vi "Acquire Data.vi"() -> ()   [LabVIEW 2020]
uses:
  states.ctl
  <vilib>/FPGAPlugInAG/cRIO-9066/niLvFpga_Open_cRIO-9066.vi
  <vilib>/rvi/interface/common/dynamic/niFpgaDynamicAddResources.vi
  <vilib>/Utility/error.llb/Error Cluster From Error Code.vi
  <vilib>/rvi/errors/niLvFpgaAdjustHostInterfaceError.vi
  <vilib>/rvi/interface/nirviOpenFPGA/nirviOpenFPGA.xnode
  FPGA Bitfiles/realcrioexample_FPGATarget_GetcRIOTemp_ZmXcEI1H0PA.lvbitx
  FPGA/Get cRIO Temp.vi
  <vilib>/rvi/interface/nirviReadWriteControl/nirviReadWriteControl.xnode
  NiFpgaLv.dll
  <vilib>/rvi/interface/Simulation/niFpgaSimulationCallBeginRW.vi
panel:
  out "Chassis Temperature":i16
  out "Chassis Temp History":i16[](array[numeric])
  in  "shutdown":bool
  in  "save to txt":bool
  in  "grab cRIO data":bool
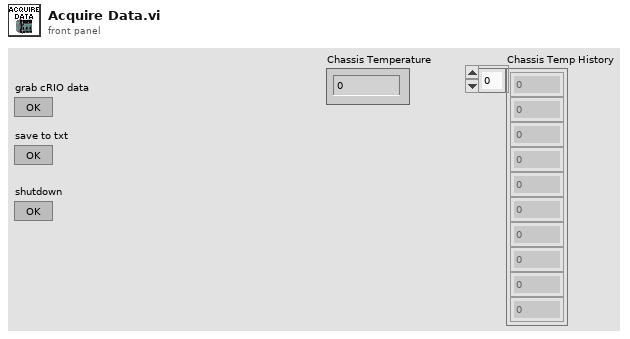
[diagram p1: front panel]
types:
  T1 = typedef "states.ctl" = enum16{"Start", "Save Data", "Shutdown"}
  T2 = enum16{"open", "replace", "create", "open or create", "replace or create", "replace or create with confirmation"}
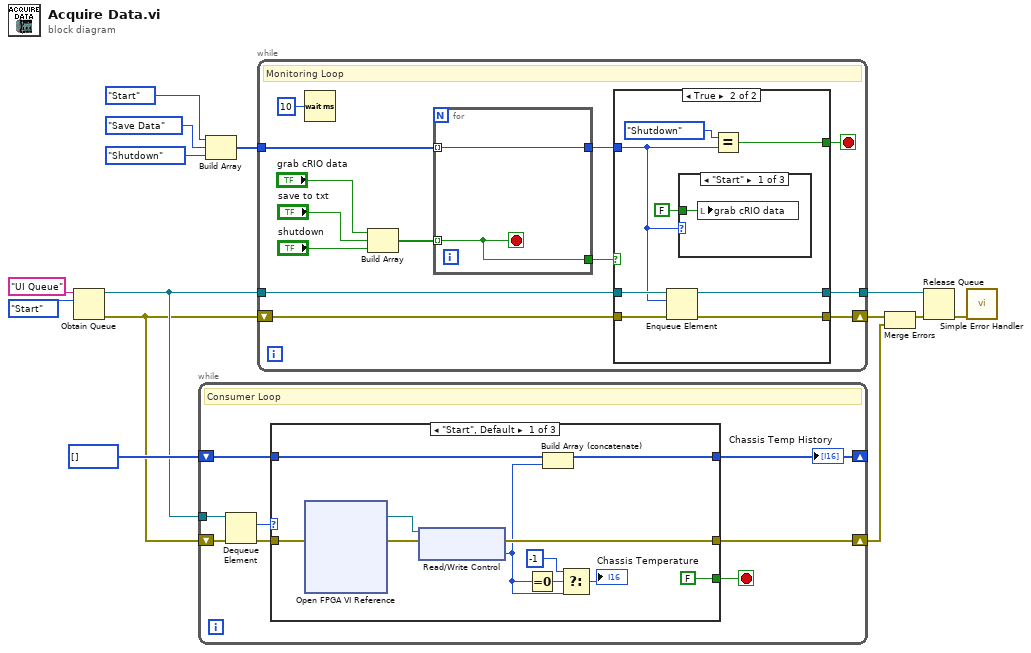
[diagram p0: block diagram]
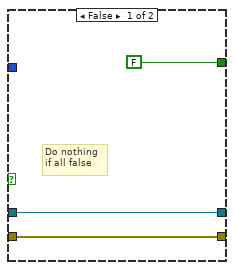
[diagram p2: hidden frame]
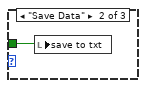
[diagram p3: hidden frame]
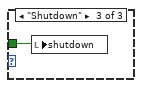
[diagram p4: hidden frame]
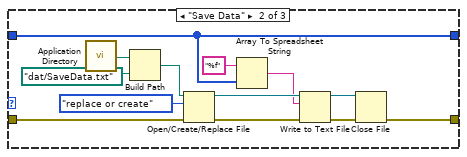
[diagram p5: hidden frame]
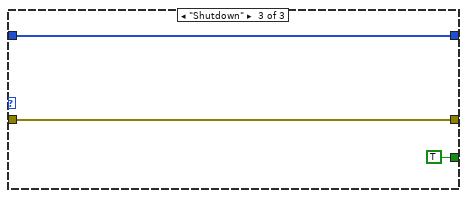
[diagram p6: hidden frame]
diagram:
  n1 = Obtain Queue(name (unnamed)="UI Queue", element data type=states."Start") -> (queue out=w5:refnum<queue>, error out=w4:errorcluster)  [unwired: 3 in, 1 out]
  n2 = while {
    tunnel: w5 -> [w22]
    shift-right: [w18] -> _
    shift-left: i16[] [] -> [w17]
    shift-right: [w15] -> w10
    shift-left: w4 -> [w21]
    stop <- w19 stop-if-true
    # "Consumer Loop"
    n3 = Dequeue Element(queue=w22, error in (no error)=w21) -> (element=w20:T1, error out=w16:errorcluster)  [unwired: 1 in, 2 out]
    n4 = case shown="\"Start\", Default" w20 {
      tunnel: [FALSE _ TRUE] -> w19
      tunnel: [w27 w45 w49] -> w18
      tunnel: w17 -> [w28 w45 w49]
      tunnel: w16 -> [w32 w35 w48]
      tunnel: [w29 w34 w48] -> w15
      frame "Start", Default {
        n5 = xnode "Open FPGA VI Reference"("error in"=w32) -> ("FPGA VI Reference Out"=w31:refnum<k20>, "error out"=w30:errorcluster)  [unwired: 1 in]
        n6 = xnode "Read/Write Control"("FPGA VI Reference In"=w31, "error in"=w30) -> ("error out"=w29:errorcluster, "chassis temp"=w23:i16)  [unwired: 1 out]
        n7 = Equal To 0?(x=w23) -> (x = 0?=w26:bool)
        n8 = Build Array (concatenate)(w28, w23) -> (w27:i16[])
        n9 = Select(t=i16 -1 ("f"), s=w26, f=w23) -> (s? t:f=→"Chassis Temperature":i16)
      }
      frame "Save Data" {
        n10 = call <vilib>:"Application Directory.vi"() -> ("Application Directory"=w38:path)
        n11 = Build Path(base path=w38, name or relative path=path "dat/SaveData.txt") -> (appended path=w36:path)
        n12 = Open/Create/Replace File(file path (use dialog)=w36, error in=w35, operation (0:open)=T2."replace or create") -> (refnum out=w43:refnum<file>, error out=w41:errorcluster)  [unwired: 3 in, 1 out]
        n13 = Array To Spreadsheet String(array=w45, 3:"%f" ("format string")) -> (spreadsheet string=w42:string)  [unwired: 1 in]
        n14 = Write to Text File(file (use dialog)=w43, text=w42, error in=w41) -> (refnum out=w40:refnum<file>, error out=w39:errorcluster)  [unwired: 1 in, 1 out]
        n15 = Close File(refnum=w40, error in=w39) -> (error out=w34:errorcluster)  [unwired: 1 out]
      }
      frame "Shutdown" {
      }
    }
    "Chassis Temp History" <- w18
  }
  n16 = Build Array(states."Start", states."Save Data", states."Shutdown") -> (w6:T1[])
  n17 = while {
    tunnel: w6 -> [w58]
    tunnel: w5 -> [w55]
    shift-right: [w52] -> w3
    shift-left: w4 -> [w53]
    tunnel: [w51] -> w2
    stop <- w50 stop-if-true
    # "Monitoring Loop"
    n18 = Wait (ms)(milliseconds to wait=u32 10) -> ()  [unwired: 1 out]
    n19 = Build Array("grab cRIO data", "save to txt", "shutdown") -> (w57:bool[])
    n20 = for {
      tunnel: w58 -> [w78] mode=indexing
      tunnel: w57 -> [w77] mode=indexing
      tunnel: [w78] -> w54
      tunnel: [w77] -> w56
      stop <- w77 stop-if-true
    }
    n21 = case shown="True" w56 {
      tunnel: w55 -> [w64 w73]
      tunnel: w54 -> [_ w67]
      tunnel: w53 -> [w65 w72]
      tunnel: [w65 w71] -> w52
      tunnel: [w64 w70] -> w51
      tunnel: [FALSE w68] -> w50
      frame False {
        # "Do nothing if all false"
      }
      frame True {
        n22 = Enqueue Element(queue=w73, element=w67, error in (no error)=w72) -> (queue out=w70:refnum<queue>, error out=w71:errorcluster)  [unwired: 1 in, 1 out]
        n23 = case shown="\"Start\"" w67 {
          tunnel: FALSE ("grab cRIO data") -> [w74 w75 w76]
          frame "Start" {
            n24 = local write "grab cRIO data"(w74) -> ()
          }
          frame "Save Data" {
            n25 = local write "save to txt"(w75) -> ()
          }
          frame "Shutdown" {
            n26 = local write "shutdown"(w76) -> ()
          }
        }
        n27 = Equal?(x=states."Shutdown", y=w67) -> (x = y?=w68:bool)
      }
    }
  }
  n28 = Merge Errors(w3, w10) -> (w12:errorcluster)
  n29 = Release Queue(queue=w2, error in (no error)=w12) -> (error out=w1:errorcluster)  [unwired: 1 in, 2 out]
  n30 = call <vilib>:"Simple Error Handler.vi"("error in (no error)"=w1) -> ()  [unwired: 4 in, 5 out]
